vi "Zero Crossing Finder.vi"(4 "dX/dt":dbl[](array[numeric])) -> (1 "Array":bool[](array[boolean]))   [LabVIEW 2013]
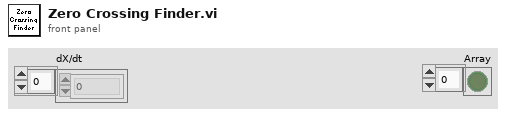
[diagram p1: front panel]
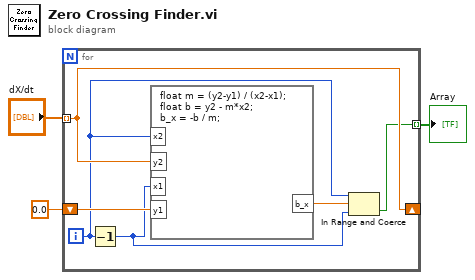
[diagram p0: block diagram]
diagram:
  n1 = for {
    shift-right: [w8] -> _
    shift-left: 0.0 -> [w9]
    tunnel: "dX/dt" -> [w8] mode=indexing
    tunnel: [w5] -> w1 mode=indexing
    i -> [w6]
    n2 = Decrement(x=w6) -> (x-1=w7:i32)
    n3 = formula code="float m = (y2-y1) / (x2-x1);\nfloat b = y2 - m*x2;\nb_x = -b / m;"("x2"=w6, "y2"=w8, "x1"=w7, "y1"=w9) -> ("b_x"=w4:dbl)
    n4 = In Range and Coerce(upper limit=w6, x=w4, lower limit=w7) -> (In Range?=w5:bool)  [unwired: 1 out]
  }
  "Array" <- w1
